vi "Generate Comments.vi"(0 "Ring in":refnum<vi>, 1 "Cluster":T3, 5 "error in (no error)":errorcluster) -> (14 "Comments":string, 19 "error out":errorcluster)   [LabVIEW 2016, in "Transport.lvclass"]
uses:
  Transport.lvclass
  <userlib>/LevyLab/Krohn Hite 7008/typedefs/Gain-Enum.ctl
  <userlib>/LevyLab/Krohn Hite 7008/typedefs/Shunt-Enum.ctl
  <userlib>/LevyLab/Krohn Hite 7008/KH7008.lvclass
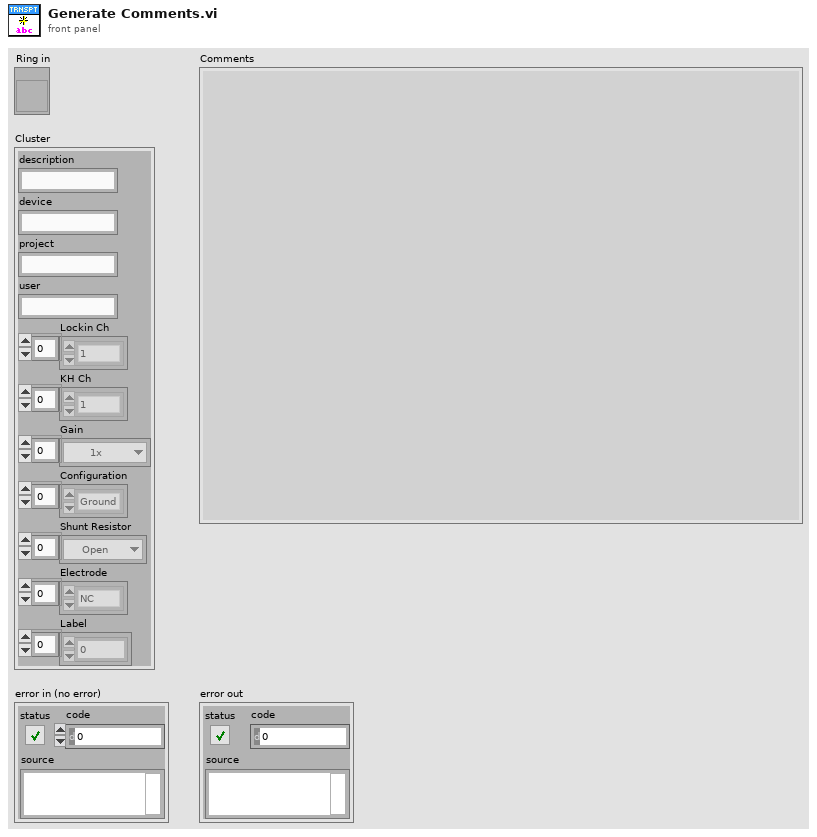
[diagram p1: front panel]
types:
  T1 = typedef "KH7008.lvclass/Gain-Enum.ctl" = enum16{"1x", "10x", "100x", "1000x"}
  T2 = typedef "KH7008.lvclass/Shunt-Enum.ctl" = enum16{"Open", "50 Ohms", "500 Ohms", "5k Ohms", "50k Ohms"}
  T3 = cluster{"description":string, "device":string, "project":string, "user":string, "Lockin Ch":enum16{"1", "2", "3", "4", "5", "6", "7", "8"}[], "KH Ch":enum16{"1", "2", "3", "4", "5", "6", "7", "8"}[], "Gain":T1[], "Configuration":enum16{"Ground", "Current", "Voltage", "Gate"}[], "Shunt Resistor":T2[], "Electrode":enum16{"NC", "26", "27", "28", "1", "2", "3", "4", "5", "6", "7", "8", "9", "10", "11", "12", "13", "14", "15", "16", "17", "18", "19", "20", "21", "22", "23", "24", "25"}[], "Label":u16[]}
  T4 = enum16{"NC", "26", "27", "28", "1", "2", "3", "4", "5", "6", "7", "8", "9", "10", "11", "12", "13", "14", "15", "16", "17", "18", "19", "20", "21", "22", "23", "24", "25"}[]
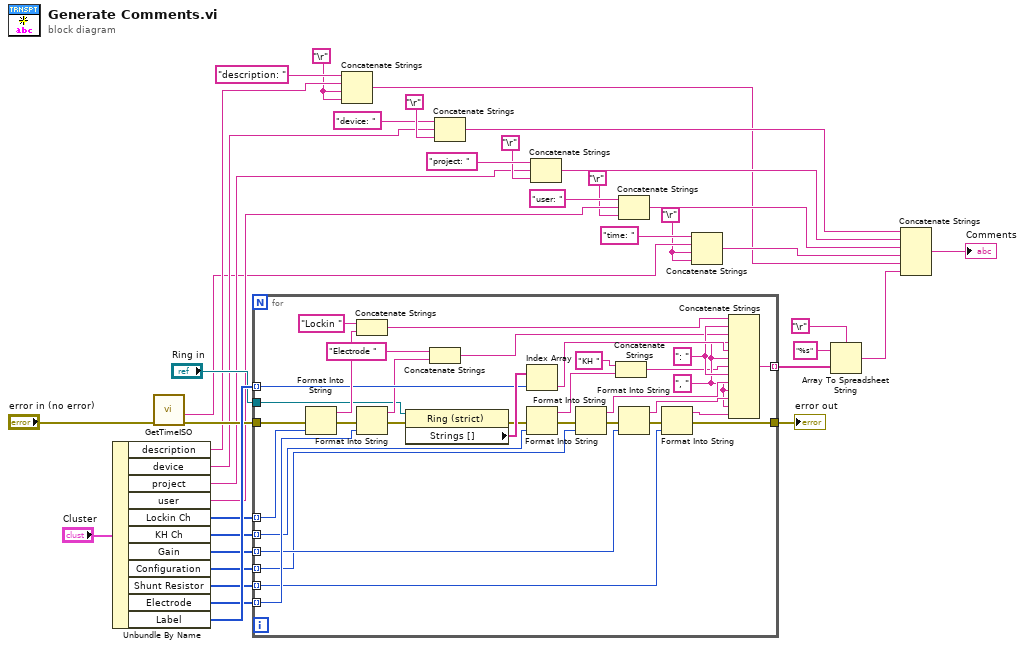
[diagram p0: block diagram]
diagram:
  w2 = "\r"
  w3 = "\r"
  n1 = Unbundle By Name("Cluster") -> ("description"=w19:string, "device"=w13:string, "project"=w12:string, "user"=w11:string, "Lockin Ch"=w31:enum16{"1", "2", "3", "4", "5", "6", "7", "8"}[], "KH Ch"=w32:enum16{"1", "2", "3", "4", "5", "6", "7", "8"}[], "Gain"=w33:T1[], "Configuration"=w34:enum16{"Ground", "Current", "Voltage", "Gate"}[], "Shunt Resistor"=w35:T2[], "Electrode"=w36:T4, "Label"=w37:u16[])
  n2 = call "GetTimeISO.vi"("error in (no error)"="error in (no error)") -> ("error out"=w22:errorcluster, "ISO 8601 date-time string"=w8:string)  [unwired: 8 in, 1 out]
  n3 = for {
    tunnel: w31 -> [w70] mode=indexing
    tunnel: w32 -> [w47] mode=indexing
    tunnel: w33 -> [w59] mode=indexing
    tunnel: w34 -> [w57] mode=indexing
    tunnel: w35 -> [w52] mode=indexing
    tunnel: w36 -> [w61] mode=indexing
    tunnel: w37 -> [w63] mode=indexing
    tunnel: [w65] -> w24 mode=indexing
    tunnel: "Ring in" -> [w46]
    tunnel: w22 -> [w45]
    tunnel: [w38] -> w21
    w54 = ", "
    w58 = ": "
    n4 = Format Into String(error in=w45, w70) -> (resulting string=w68:string, error out=w44:errorcluster)  [unwired: 2 in]
    n5 = Concatenate Strings("Lockin ", w68) -> (w66:string)
    n6 = Format Into String(error in=w44, w61) -> (resulting string=w60:string, error out=w43:errorcluster)  [unwired: 2 in]
    n7 = property on="Property Node" class="Ring (strict)"(reference=w46, error in=w43) -> (error out=w42:errorcluster, "Strings []"=w64:string[])  [unwired: 1 out]
    n8 = Concatenate Strings("Electrode ", w60) -> (w50:string)
    n9 = Index Array(array=w64, index=w63) -> (element=w62:string)
    n10 = Format Into String(error in=w42, w47) -> (resulting string=w48:string, error out=w41:errorcluster)  [unwired: 2 in]
    n11 = Format Into String(error in=w41, w57) -> (resulting string=w56:string, error out=w40:errorcluster)  [unwired: 2 in]
    n12 = Concatenate Strings("KH ", w48) -> (w49:string)
    n13 = Format Into String(error in=w40, w59) -> (resulting string=w55:string, error out=w39:errorcluster)  [unwired: 2 in]
    n14 = Format Into String(error in=w39, w52) -> (resulting string=w53:string, error out=w38:errorcluster)  [unwired: 2 in]
    n15 = Concatenate Strings(w66, w58, w50, w54, w62, w54, w49, w58, w56, w54, w55, w54, w53) -> (w65:string)
  }
  "error out" <- w21
  n16 = Concatenate Strings("description: " ("string"), w19, w3, w3) -> (w1:string)
  n17 = Concatenate Strings("device: " ("string"), w13, "\r") -> (w7:string)
  n18 = Concatenate Strings("project: " ("string"), w12, "\r") -> (w6:string)
  n19 = Concatenate Strings("user: " ("string"), w11, "\r") -> (w5:string)
  n20 = Concatenate Strings("time: " ("string"), w8, w2, w2) -> (w4:string)
  n21 = Array To Spreadsheet String(delimiter (Tab)="\r", array=w24, 3:"%s" ("format string")) -> (spreadsheet string=w27:string)
  n22 = Concatenate Strings(w7, w6, w5, w4, w1, w27) -> (→"Comments":string)
